vi "LJM_FLOAT32ToByteArray.vi"(1 "Float":sgl format="%.6f") -> (0 "Byte Array":u8[](array[numeric]))   [LabVIEW 2020]
panel:
  # "Converts a single-precision float to a big-endian byte array"
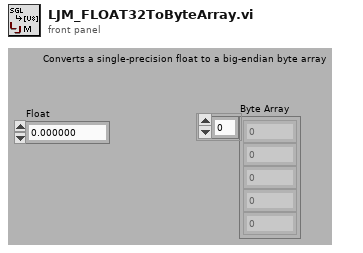
[diagram p1: front panel]
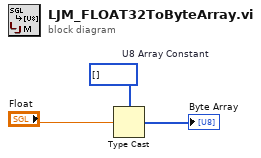
[diagram p0: block diagram]
diagram:
  w2 = u8[] []  # U8 Array Constant
  n1 = Type Cast(type=w2, x="Float") -> (*(type *) &x=→"Byte Array":u8[])
